vi "LtaSetModuleProperties.vi"(8 "Error In":errorcluster[](array[cluster]), 9 "XmlData":string, 10 "Arg":string, 11 "Test.lvclass":refnum<class "Test.lvclass">) -> (0 "Error Out":errorcluster[](array[cluster]), 3 "Test.lvclass":refnum<class "Test.lvclass">)   [LabVIEW 2018, in "Test.lvclass"]
doc: "Sets a property of one or more plugins that are currently running."
uses:
  Test.lvclass
  Test.lvclass/Test.ctl
  Sync/SyncPlugins/SyncPluginBase/Typedefs/clTimedTrigger.ctl
  Sync/SyncPlugins/PXI_MultiTrig/Typedefs/clClocks.ctl
  FGen/MemberClasses/PmuTestFunctions/Typedefs/PmuFcnArbs.ctl
  Analysis/AnalysisPlugins/FitterBaseClass/Typedefs/clAnalysisConfig.ctl
  Accessors/Read ModuleIDs.vi
  Accessors/Read ErrorSeverity.vi
  <vilib>/Utility/error.llb/Error Cluster From Error Code.vi
  <vilib>/ErrorRing/Error Ring.xnode
  Sync/SyncPlugins/SyncPluginBase/SyncPluginBase.lvclass
  <userlib>/NIST/NISTErrorLib/NISTErrorLib.lvlib
  FGen/FgenPlugins/FgenPluginBaseClass/FgenPluginsBase.lvclass
  AcPwr/AcPwrModule/AcPwrModule.lvlib
  Sync/SyncPlugins/PXI_MultiTrig/PXI_MultiTrig.lvclass
  Analysis/AnalysisPlugins/FitterBaseClass/FitterBase.lvclass
  Analysis/AnalysisPlugins/AnalysisPluginBaseClass/AnalysisPluginsBase.lvclass
  Sensor/SensorModule/SensorModule.lvlib
  FGen/MemberClasses/PmuTestFunctions/PmuTestFunctions.lvclass
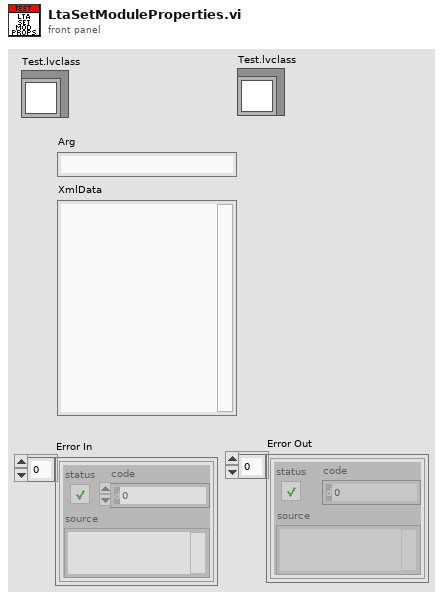
[diagram p1: front panel]
types:
  T1 = typedef "SyncPlugins.lvlib/SyncPluginBase.lvclass/clTimedTrigger.ctl" = cluster{"TriggerName":string, "Time after next UTC Second":dbl, "Trigger Duration":dbl, "Edge":enum16{"Rising", "Falling"}}
  T2 = typedef "SyncPlugins.lvlib/PXI_MultiTrig.lvclass/clClocks.ctl" = cluster{"Name":string, "RefClk":string, "ClkTerminal":string, "Frequency":dbl, "DutyCycle":dbl, "ClkType":string, "Initiated":bool, "TrigTime":bool, "Delay":dbl}
  T3 = typedef "Functions.lvlib/PmuTestFunctions.lvclass/PmuFcnArbs.ctl" = cluster{"Arbs":cluster{"Handle":string, "Size":i32, "Gain":dbl, "Offset":dbl}[], "SampleRate":dbl, "SettlingTime":dbl, "T0":dbl}
  T4 = typedef "AnalysisPlugins.lvlib/FitterBase.lvclass/clAnalysisConfig.ctl" = cluster{"F0":u32, "SettlingTime":dbl, "AnalysisCycles":dbl, "SampleRate":dbl, "NumChannels":u32, "TsOffset":enum16{"start", "middle", "end"}}
  T5 = cluster{"F0":u32, "SettlingTime":dbl, "AnalysisCycles":dbl, "SampleRate":dbl, "NumChannels":u32}
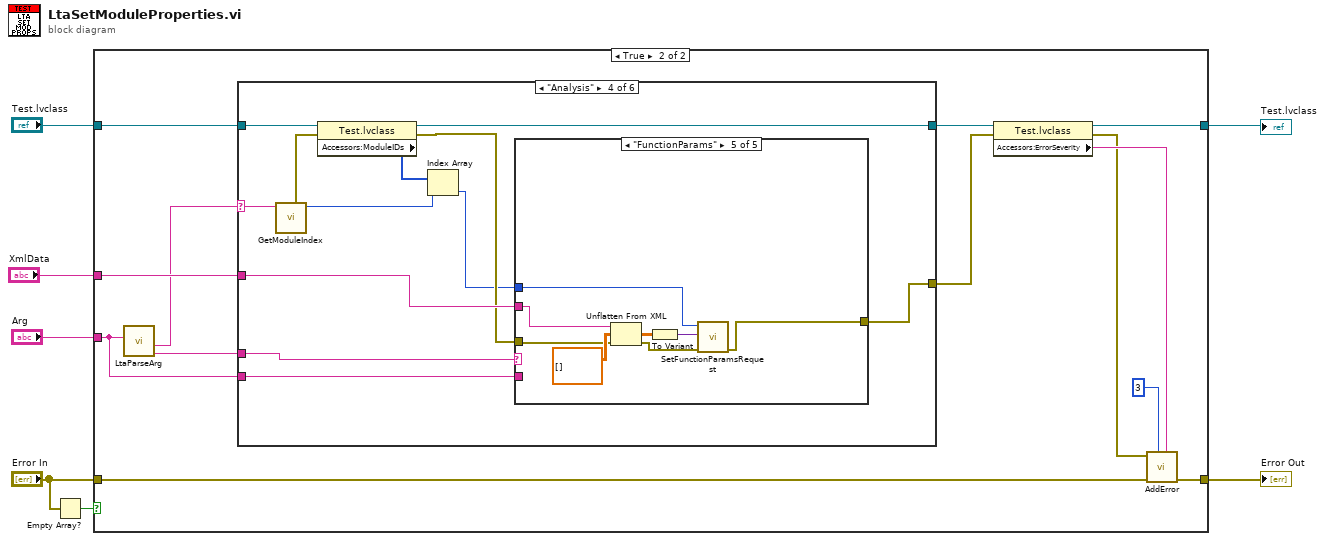
[diagram p0: block diagram]
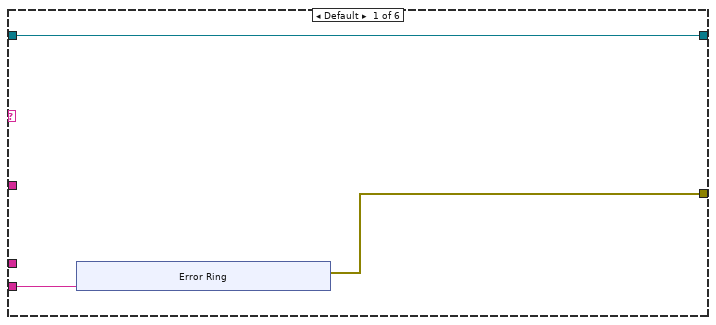
[diagram p3: hidden frame]
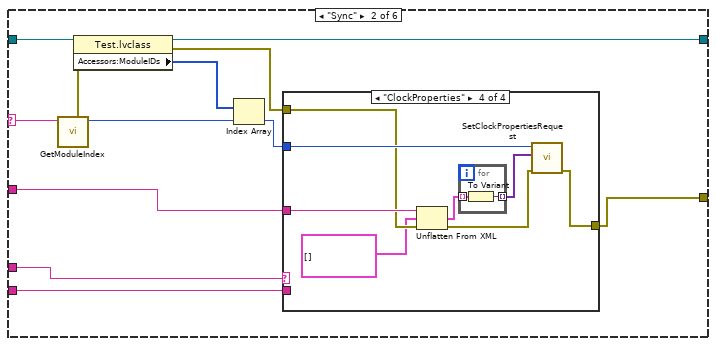
[diagram p4: hidden frame]
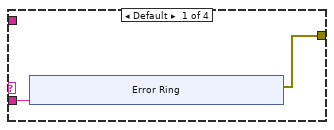
[diagram p5: hidden frame]
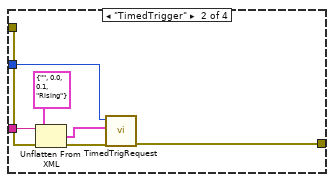
[diagram p6: hidden frame]
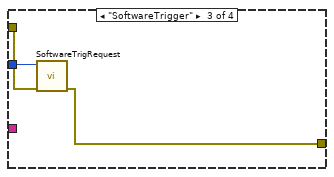
[diagram p7: hidden frame]
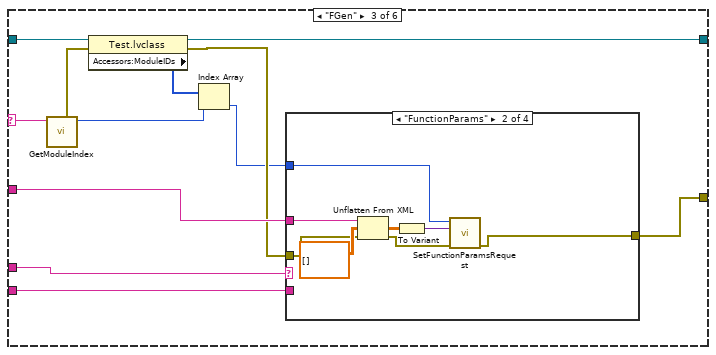
[diagram p8: hidden frame]
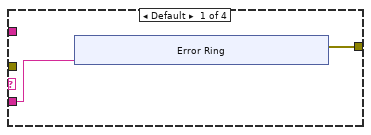
[diagram p9: hidden frame]
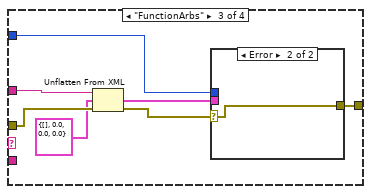
[diagram p10: hidden frame]
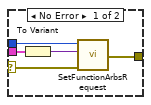
[diagram p11: hidden frame]
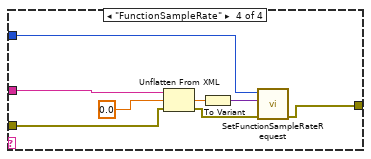
[diagram p12: hidden frame]
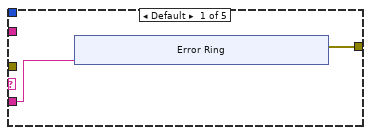
[diagram p13: hidden frame]
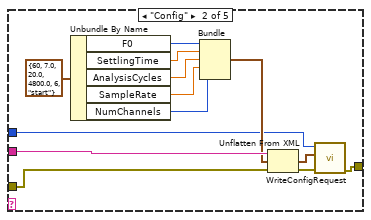
[diagram p14: hidden frame]
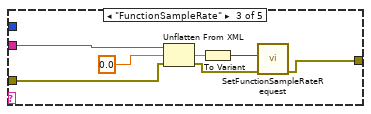
[diagram p15: hidden frame]
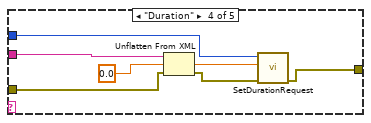
[diagram p16: hidden frame]
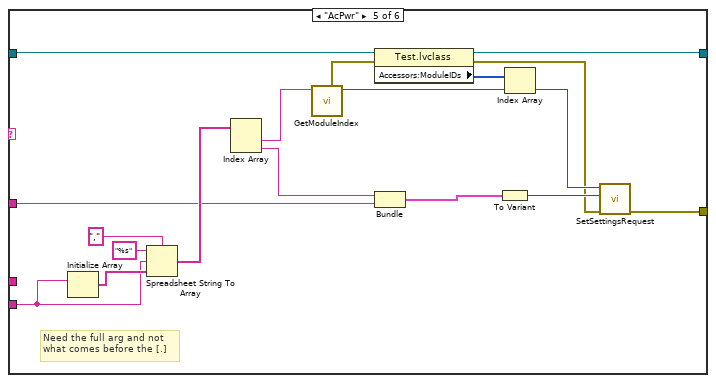
[diagram p17: hidden frame]
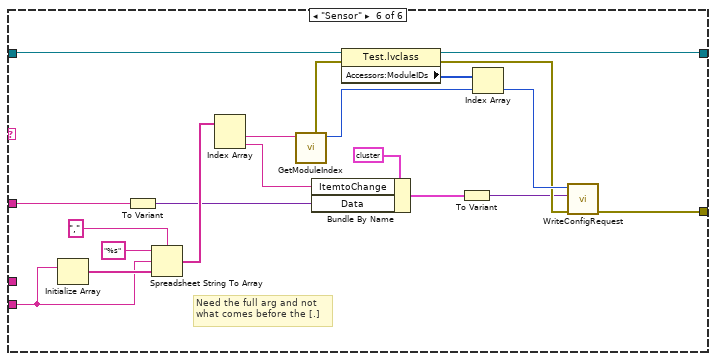
[diagram p18: hidden frame]
diagram:
  n1 = Empty Array?(array="Error In") -> (empty?=w7:bool)
  n2 = case shown="True" w7 {
    tunnel: "Error In" -> [w9 w16]
    tunnel: [w9 w19] -> w5
    tunnel: [w8 w15] -> w3
    tunnel: "Test.lvclass" -> [w8 w11]
    tunnel: "Arg" -> [_ w21]
    tunnel: "XmlData" -> [_ w20]
    frame False {
    }
    frame True {
      n3 = call "LtaParseArg.vi"("Arg In"=w21) -> ("ArgRemaining"=w22:string, "Arg 1"=w10:string)  [unwired: 8 in, 1 out]
      n4 = case shown="\"Analysis\"" w10 {
        selector: w10 -> [_ w34 w78 w128 _ _]
        tunnel: w22 -> [_ w44 w85 w135 _ _]
        tunnel: w21 -> [w25 w43 w83 w133 w184 w212]
        tunnel: w20 -> [_ w42 w82 w132 w181 w208]
        tunnel: [w24 w41 w84 w134 w192 w209] -> w14
        tunnel: w11 -> [w23 w35 w77 w127 w194 w217]
        tunnel: [w23 w33 w76 w126 w193 w216] -> w12
        frame Default {
          n5 = xnode "Error Ring"("parameter 0"=w25) -> ("error out"=w24:errorcluster)
        }
        frame "Sync" {
          n6 = call "GetModuleIndex.vi"("ModuleType"=w34) -> ("ModuleIndex"=w39:i32, "Error"=w38:errorcluster)  [unwired: 9 in]
          n7 = property class="Test.lvclass"(reference=w35, error in=w38) -> (reference out=w33:refnum<class "Test.lvclass">, error out=w36:errorcluster, "Accessors:ModuleIDs"=w40:i32[])
          n8 = Index Array(array=w40, index=w39) -> (element=w37:i32)
          n9 = case shown="\"ClockProperties\"" w44 {
            tunnel: w43 -> [w46 _ _ _]
            tunnel: w42 -> [_ w60 _ w71]
            tunnel: w36 -> [_ w55 w62 w69]
            tunnel: w37 -> [_ w56 w63 w70]
            tunnel: [w45 w54 w61 w64] -> w41
            frame Default {
              n10 = xnode "Error Ring"("parameter 0"=w46) -> ("error out"=w45:errorcluster)
            }
            frame "TimedTrigger" {
              n11 = Unflatten From XML(xml string=w60, type=T1 {"TriggerName"="", "Time after next UTC Second"=0.0, "Trigger Duration"=0.1, "Edge"=enum."Rising"} ("clTimedTrigger"), error in (no error)=w55) -> (value=w57:T1, error out=w58:errorcluster)
              n12 = call "TimedTrigRequest.vi"("error in (no error)"=w58, "Time after next UTC Second"=w57, "ModuleID"=w56) -> ("error out"=w54:errorcluster)  [unwired: 8 in]
            }
            frame "SoftwareTrigger" {
              n13 = call "SoftwareTrigRequest.vi"("error in (no error)"=w62, "ModuleID"=w63) -> ("error out"=w61:errorcluster)  [unwired: 9 in]
            }
            frame "ClockProperties" {
              n14 = Unflatten From XML(xml string=w71, type=T2[] [], error in (no error)=w69) -> (value=w67:T2[], error out=w65:errorcluster)
              n15 = for {
                tunnel: w67 -> [w73] mode=indexing
                tunnel: [w72] -> w66 mode=indexing
                n16 = To Variant(anything=w73) -> (Variant=w72:variant)
              }
              n17 = call "SetClockPropertiesRequest.vi"("error in (no error)"=w65, "ClockProperties"=w66, "ModuleID"=w70) -> ("error out"=w64:errorcluster)  [unwired: 8 in]
            }
          }
        }
        frame "FGen" {
          n18 = call "GetModuleIndex.vi"("ModuleType"=w78) -> ("ModuleIndex"=w80:i32, "Error"=w79:errorcluster)  [unwired: 9 in]
          n19 = property class="Test.lvclass"(reference=w77, error in=w79) -> (reference out=w76:refnum<class "Test.lvclass">, error out=w75:errorcluster, "Accessors:ModuleIDs"=w81:i32[])
          n20 = Index Array(array=w81, index=w80) -> (element=w74:i32)
          n21 = case shown="\"FunctionParams\"" w85 {
            tunnel: [w87 w97 w106 w120] -> w84
            tunnel: w83 -> [w86 _ _ _]
            tunnel: w82 -> [_ w102 w109 w123]
            tunnel: w75 -> [_ w96 w105 w117]
            tunnel: w74 -> [_ w95 w104 w116]
            frame Default {
              n22 = xnode "Error Ring"("parameter 0"=w86) -> ("error out"=w87:errorcluster)
            }
            frame "FunctionParams" {
              n23 = Unflatten From XML(xml string=w102, type=dbl[][] [], error in (no error)=w96) -> (value=w99:dbl[][], error out=w98:errorcluster)
              n24 = To Variant(anything=w99) -> (Variant=w100:variant)
              n25 = call "SetFunctionParamsRequest.vi"("error in (no error)"=w98, "FunctionConfig"=w100, "ModuleID"=w95) -> ("error out"=w97:errorcluster)  [unwired: 8 in]
            }
            frame "FunctionArbs" {
              n26 = Unflatten From XML(xml string=w109, type=T3 {"Arbs"=[], "SampleRate"=0.0, "SettlingTime"=0.0, "T0"=0.0} ("FunctionConfig"), error in (no error)=w105) -> (value=w108:T3, error out=w107:errorcluster)
              n27 = case shown="Error" w107 {
                selector: w107 -> [w113 w115]
                tunnel: w108 -> [w114 _]
                tunnel: [w112 w115] -> w106
                tunnel: w104 -> [w110 _]
                frame No Error {
                  n28 = To Variant(anything=w114) -> (Variant=w111:variant)
                  n29 = call "SetFunctionArbsRequest.vi"("error in (no error)"=w113, "FunctionArbs"=w111, "ModuleID"=w110) -> ("error out"=w112:errorcluster)  [unwired: 8 in]
                }
                frame Error {
                }
              }
            }
            frame "FunctionSampleRate" {
              n30 = Unflatten From XML(xml string=w123, type=0.0, error in (no error)=w117) -> (value=w122:dbl, error out=w121:errorcluster)
              n31 = To Variant(anything=w122) -> (Variant=w119:variant)
              n32 = call "SetFunctionSampleRateRequest.vi"("error in (no error)"=w121, "FunctionSampleRate"=w119, "ModuleID"=w116) -> ("error out"=w120:errorcluster)  [unwired: 8 in]
            }
          }
        }
        frame "Analysis" {
          n33 = call "GetModuleIndex.vi"("ModuleType"=w128) -> ("ModuleIndex"=w130:i32, "Error"=w129:errorcluster)  [unwired: 9 in]
          n34 = property class="Test.lvclass"(reference=w127, error in=w129) -> (reference out=w126:refnum<class "Test.lvclass">, error out=w125:errorcluster, "Accessors:ModuleIDs"=w131:i32[])
          n35 = Index Array(array=w131, index=w130) -> (element=w124:i32)
          n36 = case shown="\"FunctionParams\"" w135 {
            tunnel: [w137 w145 w161 w169 w172] -> w134
            tunnel: w133 -> [w136 _ _ _ _]
            tunnel: w132 -> [_ w157 w164 w171 w176]
            tunnel: w125 -> [_ w156 w158 w167 w177]
            tunnel: w124 -> [_ w146 _ w165 w173]
            frame Default {
              n37 = xnode "Error Ring"("parameter 0"=w136) -> ("error out"=w137:errorcluster)
            }
            frame "Config" {
              n38 = Unbundle By Name(T4 {"F0"=60, "SettlingTime"=7.0, "AnalysisCycles"=20.0, "SampleRate"=4800.0, "NumChannels"=6, "TsOffset"=enum."start"} ("clAnalysisConfig")) -> ("F0"=w151:u32, "SettlingTime"=w152:dbl, "AnalysisCycles"=w153:dbl, "SampleRate"=w154:dbl, "NumChannels"=w155:u32)
              n39 = Bundle("F0"=w151, "SettlingTime"=w152, "AnalysisCycles"=w153, "SampleRate"=w154, "NumChannels"=w155) -> (w149:T5)  [unwired: 1 in]
              n40 = Unflatten From XML(xml string=w157, type=w149, error in (no error)=w156) -> (value=w147:T5, error out=w148:errorcluster)
              n41 = call "WriteConfigRequest.vi"("error in (no error)"=w148, "AnalysisConfig"=w147, "ModuleID"=w146) -> ("error out"=w145:errorcluster)  [unwired: 8 in]
            }
            frame "FunctionSampleRate" {
              n42 = Unflatten From XML(xml string=w164, type=0.0, error in (no error)=w158) -> (value=w163:dbl, error out=w162:errorcluster)
              n43 = To Variant(anything=w163) -> (Variant=w160:variant)
              n44 = call "SetFunctionSampleRateRequest.vi"("error in (no error)"=w162, "FunctionSampleRate"=w160) -> ("error out"=w161:errorcluster)  [unwired: 9 in]
            }
            frame "Duration" {
              n45 = Unflatten From XML(xml string=w171, type=0.0, error in (no error)=w167) -> (value=w166:dbl, error out=w170:errorcluster)
              n46 = call "SetDurationRequest.vi"("error in (no error)"=w170, "Duration"=w166, "ModuleID"=w165) -> ("error out"=w169:errorcluster)  [unwired: 8 in]
            }
            frame "FunctionParams" {
              n47 = Unflatten From XML(xml string=w176, type=dbl[][] [], error in (no error)=w177) -> (value=w178:dbl[][], error out=w174:errorcluster)
              n48 = To Variant(anything=w178) -> (Variant=w175:variant)
              n49 = call "SetFunctionParamsRequest.vi"("error in (no error)"=w174, "FunctionParams"=w175, "ModuleID"=w173) -> ("error out"=w172:errorcluster)  [unwired: 8 in]
            }
          }
        }
        frame "AcPwr" {
          # "Need the full arg and not \nwhat comes before the [.]"
          n50 = Initialize Array(w184) -> (w185:string[])  [unwired: 1 in]
          n51 = Spreadsheet String To Array(delimiter (Tab)=",", format string="%s", spreadsheet string=w184, array type (2D Dbl)=w185) -> (array=w186:string[])
          n52 = Index Array(array=w186) -> (element #1=w188:string, element #2=w187:string)  [unwired: 2 in]
          n53 = call "GetModuleIndex.vi"("ModuleType"=w188) -> ("ModuleIndex"=w196:i32, "Error"=w195:errorcluster)  [unwired: 9 in]
          n54 = property class="Test.lvclass"(reference=w194, error in=w195) -> (reference out=w193:refnum<class "Test.lvclass">, error out=w180:errorcluster, "Accessors:ModuleIDs"=w197:i32[])
          n55 = Bundle("Arg"=w187, "XmlData"=w181) -> (w189:cluster{"Arg":string, "XmlData":string})  [unwired: 1 in]
          n56 = To Variant(anything=w189) -> (Variant=w190:variant)
          n57 = Index Array(array=w197, index=w196) -> (element=w191:i32)
          n58 = call "SetSettingsRequest.vi"("Error In"=w180, "Data"=w190, "ModuleID"=w191) -> ("Error Out"=w192:errorcluster)  [unwired: 8 in]
        }
        frame "Sensor" {
          # "Need the full arg and not \nwhat comes before the [.]"
          n59 = Initialize Array(w212) -> (w213:string[])  [unwired: 1 in]
          n60 = To Variant(anything=w208) -> (Variant=w206:variant)
          n61 = Spreadsheet String To Array(delimiter (Tab)=",", format string="%s", spreadsheet string=w212, array type (2D Dbl)=w213) -> (array=w214:string[])
          n62 = Index Array(array=w214) -> (element #1=w215:string, element #2=w207:string)  [unwired: 2 in]
          n63 = call "GetModuleIndex.vi"("ModuleType"=w215) -> ("ModuleIndex"=w204:i32, "Error"=w203:errorcluster)  [unwired: 9 in]
          n64 = Bundle By Name(cluster=cluster{"Data":variant, "ItemtoChange":string} {"Data"=variant, "ItemtoChange"=""}, "ItemtoChange"=w207, "Data"=w206) -> (w199:cluster{"Data":variant, "ItemtoChange":string})
          n65 = property class="Test.lvclass"(reference=w217, error in=w203) -> (reference out=w216:refnum<class "Test.lvclass">, error out=w201:errorcluster, "Accessors:ModuleIDs"=w205:i32[])
          n66 = To Variant(anything=w199) -> (Variant=w198:variant)
          n67 = Index Array(array=w205, index=w204) -> (element=w202:i32)
          n68 = call "WriteConfigRequest.vi"("error in (no error)"=w201, "Config"=w198, "ModuleID"=w202) -> ("error out"=w209:errorcluster)  [unwired: 8 in]
        }
      }
      n69 = property class="Test.lvclass"(reference=w12, error in=w14) -> (reference out=w15:refnum<class "Test.lvclass">, error out=w13:errorcluster, "Accessors:ErrorSeverity"=w18:string)
      n70 = call <userlib>:"AddError.vi"("Severity"=w18, "Priority"=u8 3, "ErrorArray In"=w16, "error in (no error)"=w13) -> ("ErrorArray Out"=w19:errorcluster[])  [unwired: 6 in, 1 out]
    }
  }
  "Test.lvclass" <- w3
  "Error Out" <- w5
